vi "Sender UI.vi"(8 "Error In":errorcluster, 10 "Transmission Type":T1, 11 "Transmission Data":string(combo)) -> (0 "Error Out":errorcluster)   [LabVIEW 2020, in "Sender.lvclass"]
doc: "The VI allows user to select the type of data to be send to receiver and type of transmission"
uses:
  Sender.lvclass
  Controls/Queue Operation.ctl
  Controls/User Event Operations.ctl
  Controls/Messenger Data.ctl
  Communication/Communication.lvclass
  Data/Data.lvclass
  Controls/Class DVR Ref.ctl
  Controls/Type Class Ref.ctl
  Controls/Message Type.ctl
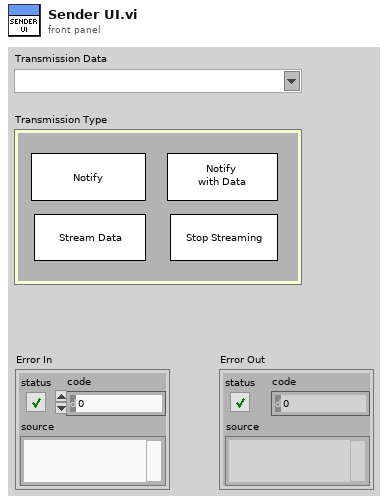
[diagram p1: front panel]
types:
  T1 = typedef "Message Type.ctl" = cluster{"Notify Only":bool, "Notify With Data":bool, "Stream Data":bool, "Stop Stream":bool}
  T2 = typedef "Messenger Data.ctl" = cluster{"Start Time":dbl, "Elapsed TIme":dbl, "Selected Data Type":string, "Selected Transmission Type":string, "Type DVR Ref":T3[], "Data DVR Ref":T4[], "Type DVR":refnum<data-value>, "Data DVR":refnum<data-value>, "Stream?":bool, "Wait Time":dbl}
  T3 = typedef "Type Class Ref.ctl" = cluster{"Class Name":string, "Class DVR Ref":refnum<data-value>}
  T4 = typedef "Class DVR Ref.ctl" = cluster{"Class DVR Ref":refnum<data-value>, "Class Name":string}
  T5 = typedef "User Event Operations.ctl" = enum16{"Obtain", "Generate", "Destroy"}
  T6 = typedef "Queue Operation.ctl" = enum16{"Create & Enqueue N", "Enqueue N", "Dequeue", "Enstack N", "Flush", "Release"}
  T7 = enum8{"Enabled", "Disabled", "Disabled and Grayed Out"}
  T8 = typedef "Queue Element.ctl" = cluster{"State":string, "Data":variant}
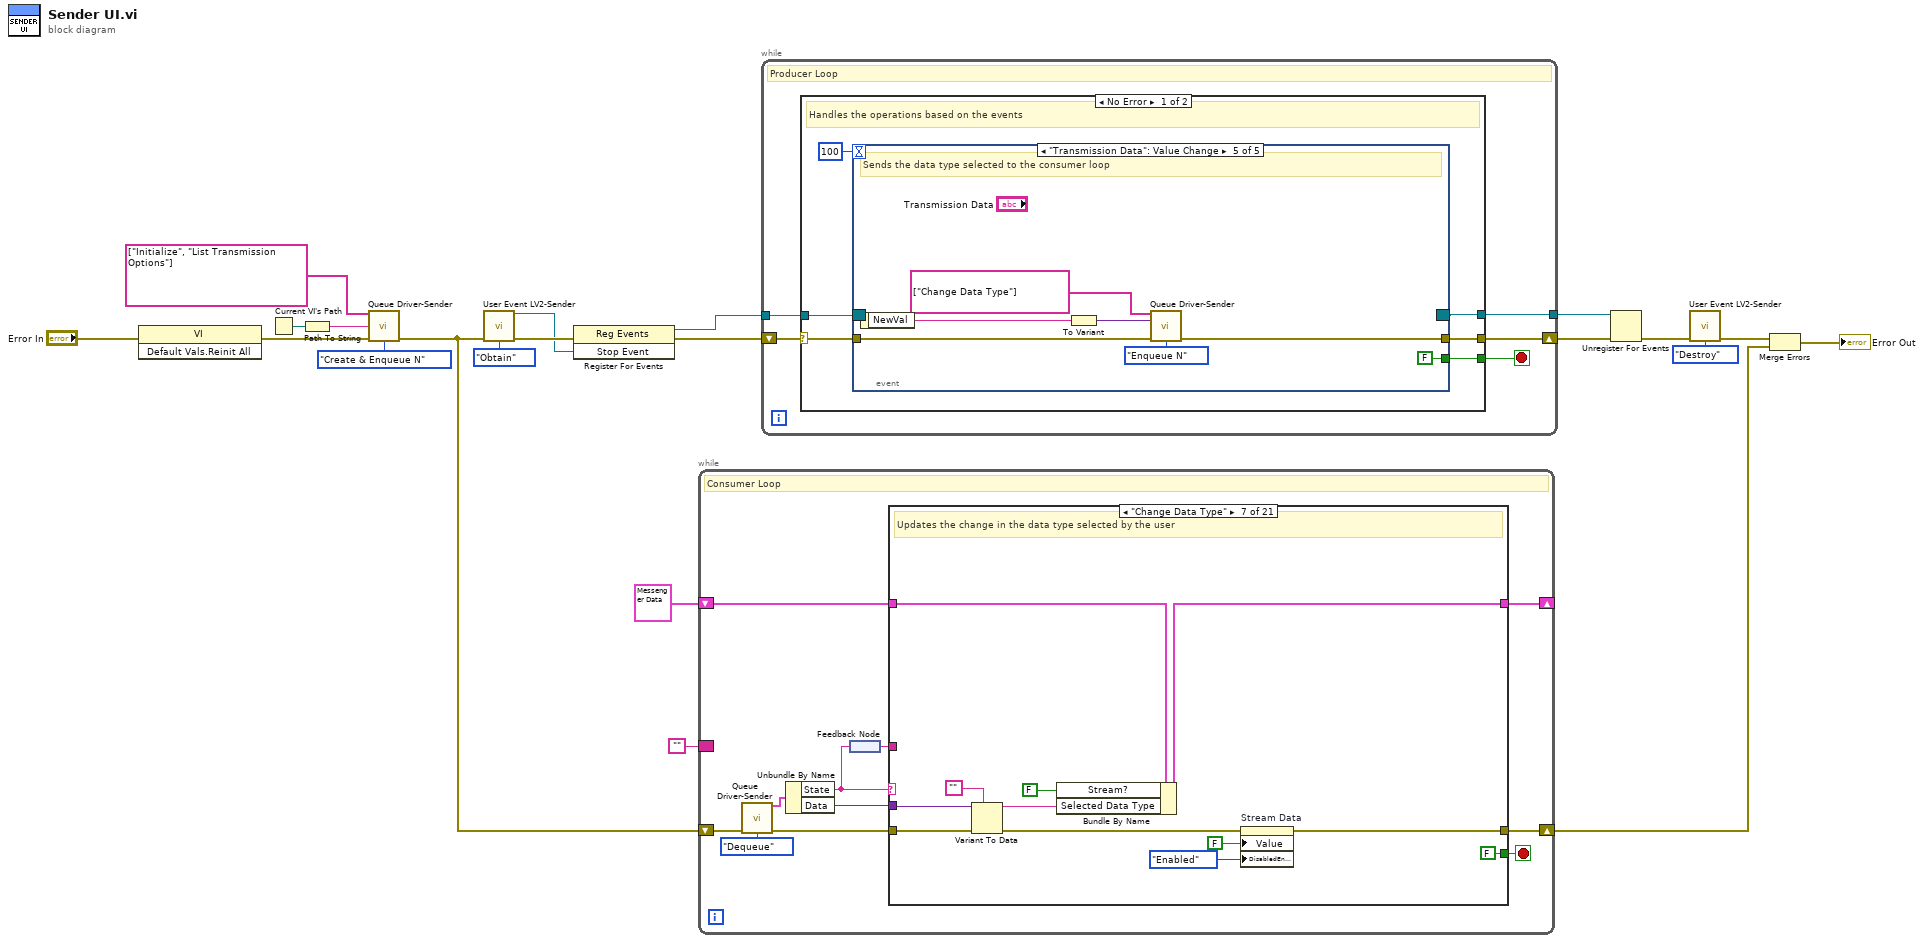
[diagram p0: block diagram]
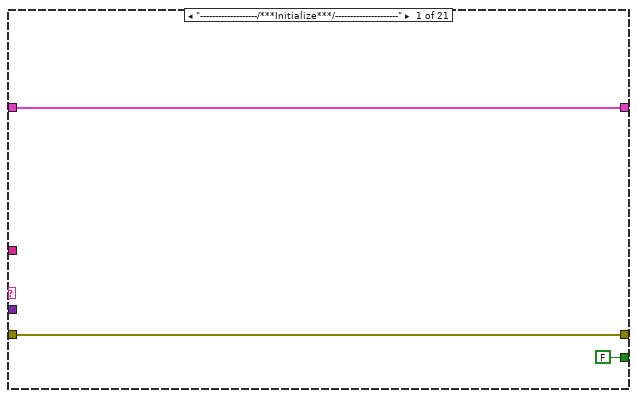
[diagram p2: hidden frame]
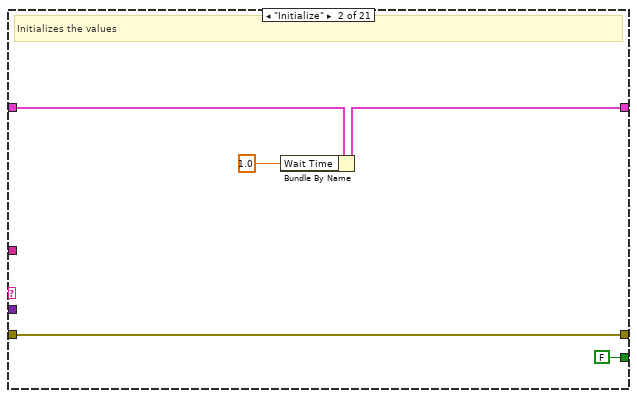
[diagram p3: hidden frame]
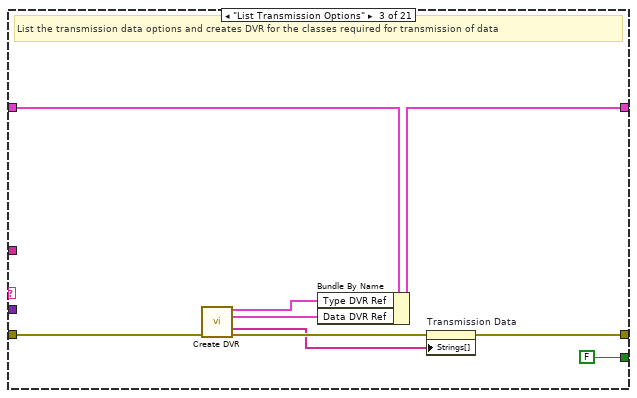
[diagram p4: hidden frame]
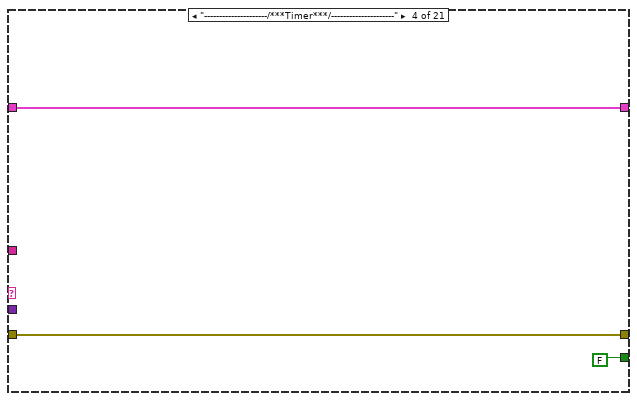
[diagram p5: hidden frame]
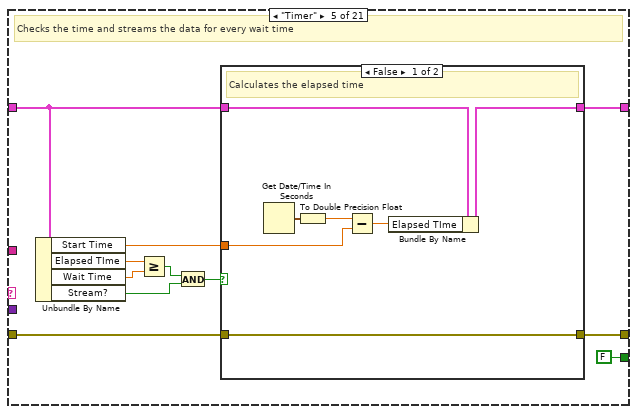
[diagram p6: hidden frame]
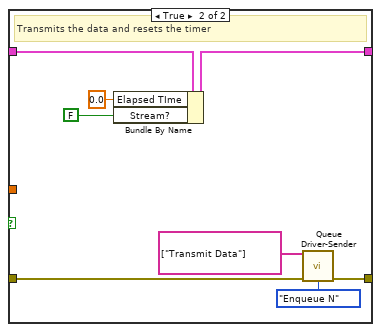
[diagram p7: hidden frame]
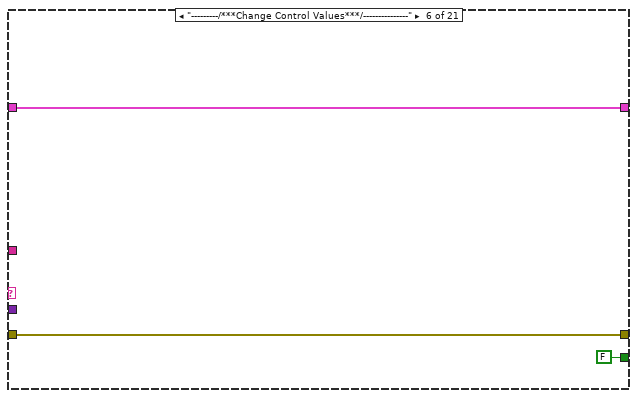
[diagram p8: hidden frame]
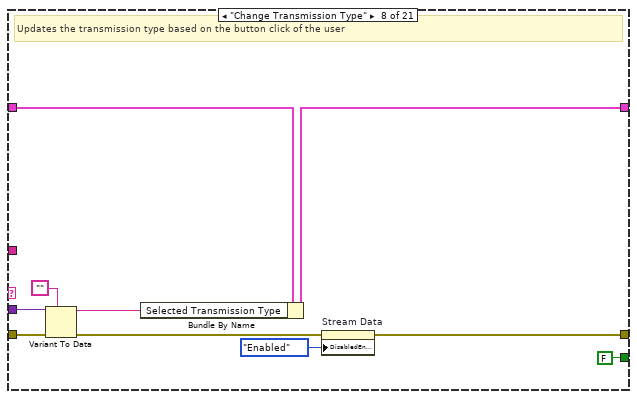
[diagram p9: hidden frame]
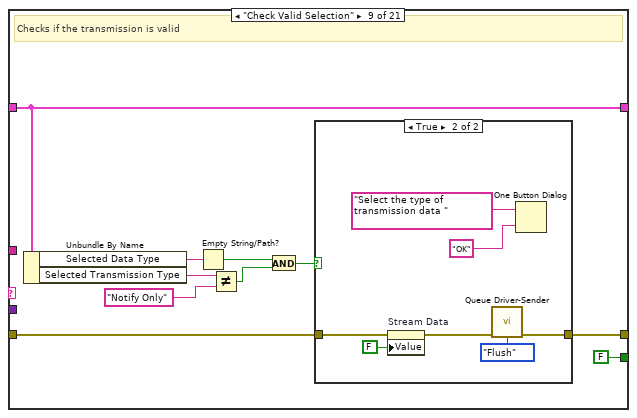
[diagram p10: hidden frame]
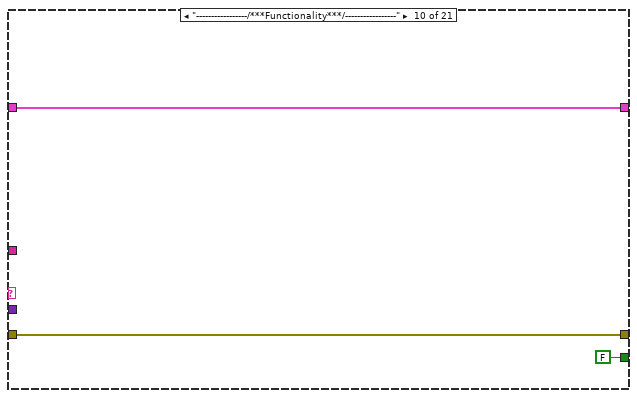
[diagram p12: hidden frame]
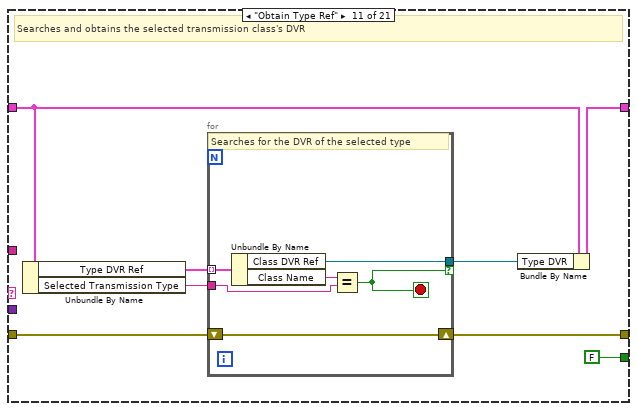
[diagram p13: hidden frame]
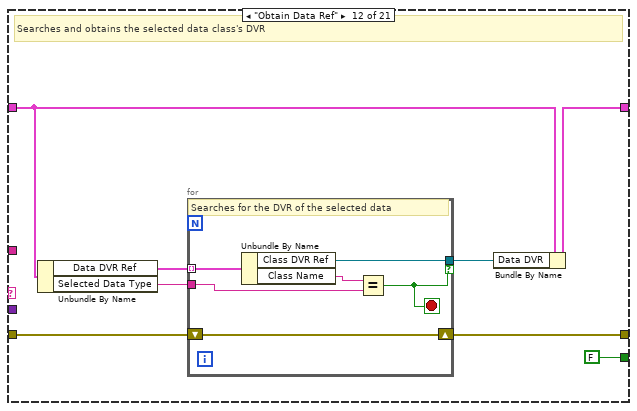
[diagram p14: hidden frame]
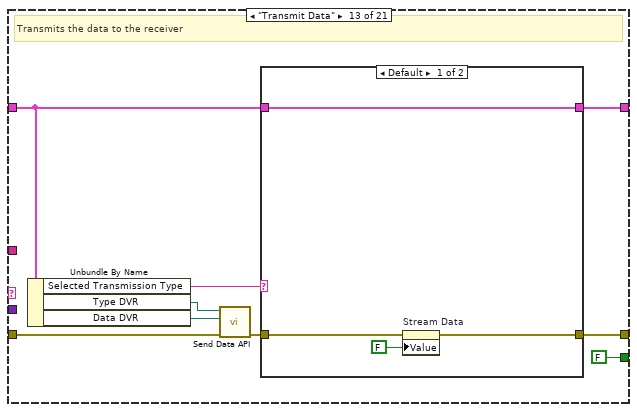
[diagram p15: hidden frame]
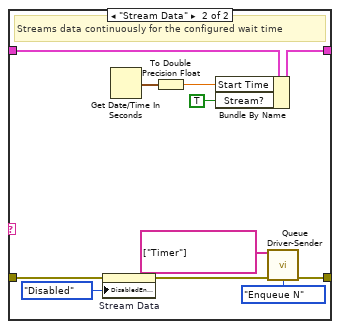
[diagram p16: hidden frame]
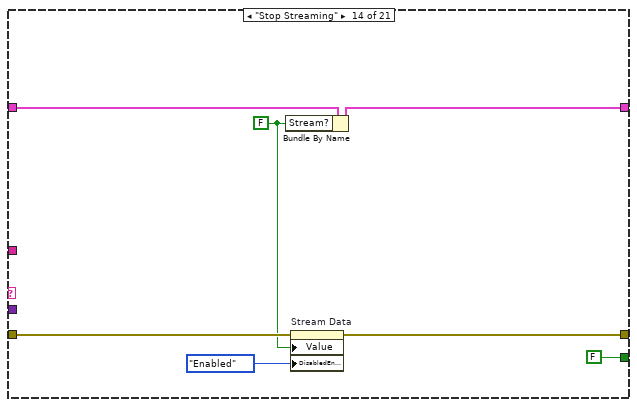
[diagram p17: hidden frame]
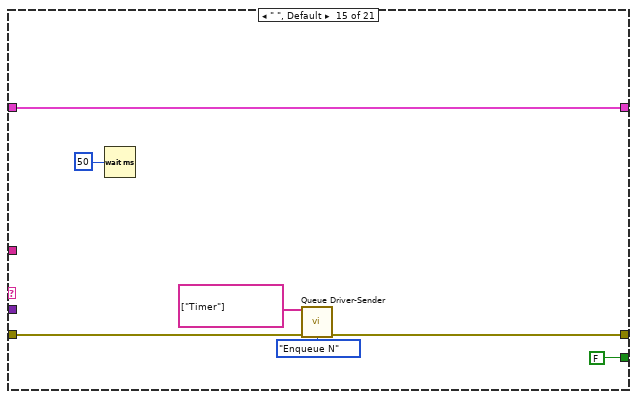
[diagram p18: hidden frame]
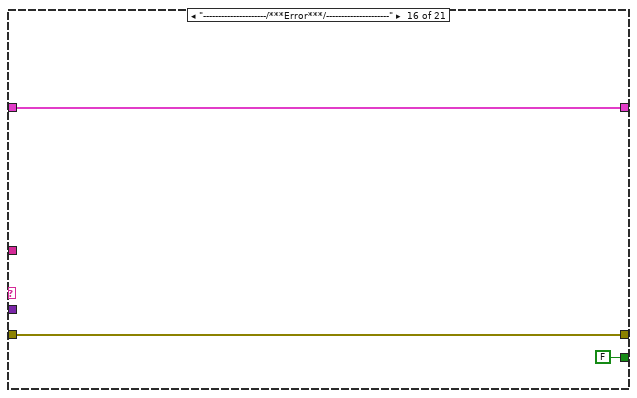
[diagram p19: hidden frame]
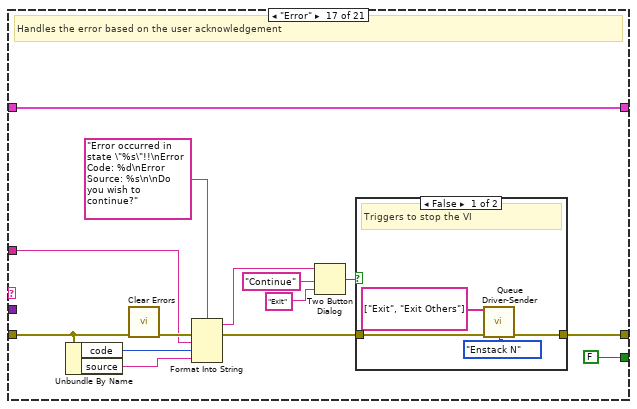
[diagram p20: hidden frame]
diagram:
  n1 = invoke class="VI" method="Default Vals.Reinit All"(error in="Error In") -> (error out=w1:errorcluster)  [unwired: 2 in, 2 out]
  n2 = Current VI's Path() -> (path=w3:path)
  n3 = Path To String(path=w3) -> (string=w2:string)
  n4 = call "Queue Driver-Sender.vi"("States[]"=string[] ["Initialize", "List Transmission Options"], "Queue Name"=w2, "Error In"=w1, "Queue Operation"=Queue_Operation."Create & Enqueue N") -> ("Error Out"=w13:errorcluster)  [unwired: 10 in, 1 out]
  n5 = call "User Event LV2-Sender.vi"("Error In"=w13, "Operation"=User_Event_Operations."Obtain") -> ("Stop Event"=w11:refnum<user-event>, "Error Out"=w15:errorcluster)  [unwired: 12 in]
  n6 = register-events(error in=w15, w11) -> (reference out=w10:refnum<event-registration>, error out=w12:errorcluster)  [unwired: 1 in]
  n7 = while {
    shift-right: [w31] -> w16
    shift-left: w13 -> [w32]
    border: "" -> [_]
    shift-right: [w22] -> _
    shift-left: T2 {"Start Time"=0.0, "Elapsed TIme"=0.0, "Selected Data Type"="", "Selected Transmission Type"="", "Type DVR Ref"=[], "Data DVR Ref"=[], "Type DVR"=refnum, "Data DVR"=refnum, "Stream?"=FALSE, "Wait Time"=0.0} -> [w23]
    stop <- w27 stop-if-true
    # "Consumer Loop"
    n8 = call "Queue Driver-Sender.vi"("Error In"=w32, "Queue Operation"=Queue_Operation."Dequeue") -> ("Dequeue Element"=w28:T8, "Error Out"=w30:errorcluster)  [unwired: 12 in]
    n9 = Unbundle By Name(w28) -> ("State"=w26:string, "Data"=w24:variant)
    n10 = feedback-in #1(w26) -> ()
    n11 = feedback #1() -> (w25:string)
    n12 = case shown="\"Change Data Type\"" w26 {
      tunnel: w30 -> [w35 w39 w49 w52 w63 w81 w93 w103 w113 w124 w132 w146 w161 w183 w190 w193 w199 w228 w236 w246 w255]
      tunnel: [w35 w39 w41 w52 w62 w81 w84 w95 w110 w124 w131 w145 w157 w179 w187 w193 w196 w215 w236 w242 w253] -> w31
      tunnel: [FALSE FALSE FALSE FALSE FALSE FALSE FALSE FALSE FALSE FALSE FALSE FALSE FALSE FALSE FALSE FALSE FALSE FALSE FALSE TRUE FALSE] -> w27
      tunnel: w25 -> [_ _ _ _ _ _ _ _ _ _ _ _ _ _ _ _ w197 _ _ _ _]
      tunnel: w24 -> [_ _ _ _ _ _ w88 w100 _ _ _ _ _ _ _ _ _ w220 _ _ _]
      tunnel: w23 -> [w33 w38 w47 w51 w60 w80 w90 w102 w111 w122 w130 w144 w156 w182 w188 w191 w194 w227 w234 w237 w254]
      tunnel: [w33 w37 w45 w51 w59 w80 w89 w98 w111 w122 w126 w140 w158 w181 w188 w191 w194 w227 w234 w237 w254] -> w22
      frame "-------------------/***Initialize***/---------------------" {
      }
      frame "Initialize" {
        # "Initializes the values"
        n13 = Bundle By Name(cluster=w38, "Wait Time"=1.0) -> (w37:T2)
      }
      frame "List Transmission Options" {
        # "List the transmission data options and creates DVR for the classes required for transmission of data"
        n14 = call "Create DVR.vi"("Error In"=w49) -> ("Communication DVR Refs"=w44:T3[], "Data Type DVR Refs"=w43:T4[], "Data Types"=w42:string[], "Error Out"=w46:errorcluster)  [unwired: 10 in, 1 out]
        n15 = Bundle By Name(cluster=w47, "Type DVR Ref"=w44, "Data DVR Ref"=w43) -> (w45:T2)
        n16 = property on="Transmission Data" class="CmbBox"(error in=w46, "Strings[]"=w42) -> (error out=w41:errorcluster)  [unwired: 1 in, 1 out]
      }
      frame "---------------------/***Timer***/---------------------" {
      }
      frame "Timer" {
        # "Checks the time and streams the data for every wait time"
        n17 = Unbundle By Name(w60) -> ("Start Time"=w61:dbl, "Elapsed TIme"=w57:dbl, "Wait Time"=w53:dbl, "Stream?"=w54:bool)
        n18 = Greater Or Equal?(x=w57, y=w53) -> (x >= y?=w56:bool)
        n19 = And(x=w56, y=w54) -> (x .and. y?=w55:bool)
        n20 = case shown="False" w55 {
          tunnel: w63 -> [w69 w71]
          tunnel: [w69 w77] -> w62
          tunnel: w61 -> [w64 _]
          tunnel: [w68 w74] -> w59
          tunnel: w60 -> [w70 w78]
          frame False {
            # "Calculates the elapsed time"
            n21 = Get Date/Time In Seconds() -> (seconds since 1Jan1904=w67:timestamp)
            n22 = To Double Precision Float(number=w67) -> (double precision float=w65:dbl)
            n23 = Subtract(x=w65, y=w64) -> (x-y=w66:dbl)
            n24 = Bundle By Name(cluster=w70, "Elapsed TIme"=w66) -> (w68:T2)
          }
          frame True {
            # "Transmits the data and resets the timer"
            n25 = Bundle By Name(cluster=w78, "Elapsed TIme"=0.0, "Stream?"=FALSE) -> (w74:T2)
            n26 = call "Queue Driver-Sender.vi"("States[]"=string[] ["Transmit Data"], "Error In"=w71, "Queue Operation"=Queue_Operation."Enqueue N") -> ("Error Out"=w77:errorcluster)  [unwired: 11 in, 1 out]
          }
        }
      }
      frame "---------/***Change Control Values***/---------------" {
      }
      frame "Change Data Type" {
        # "Updates the change in the data type selected by the user"
        n27 = Variant To Data(error in=w93, type="", Variant=w88) -> (data=w86:string, error out=w87:errorcluster)
        n28 = Bundle By Name(cluster=w90, "Stream?"=FALSE, "Selected Data Type"=w86) -> (w89:T2)
        n29 = property on="Stream Data" class="Bool (strict)"(error in=w87, "Value"=FALSE, "DisabledEnum"=T7."Enabled" ("Disabled")) -> (error out=w84:errorcluster)  [unwired: 1 in, 1 out]
      }
      frame "Change Transmission Type" {
        # "Updates the transmission type based on the button click of the user"
        n30 = Variant To Data(error in=w103, type="", Variant=w100) -> (data=w97:string, error out=w101:errorcluster)
        n31 = Bundle By Name(cluster=w102, "Selected Transmission Type"=w97) -> (w98:T2)
        n32 = property on="Stream Data" class="Bool (strict)"(error in=w101, "DisabledEnum"=T7."Enabled" ("Disabled")) -> (error out=w95:errorcluster)  [unwired: 1 in, 1 out]
      }
      frame "Check Valid Selection" {
        # "Checks if the transmission is valid"
        n33 = Unbundle By Name(w111) -> ("Selected Data Type"=w109:string, "Selected Transmission Type"=w107:string)
        n34 = Empty String/Path?(string/path=w109) -> (empty?=w106:bool)
        n35 = Not Equal?(x=w107, y="Notify Only") -> (x != y?=w105:bool)
        n36 = And(x=w106, y=w105) -> (x .and. y?=w104:bool)
        n37 = case shown="True" w104 {
          tunnel: w113 -> [w114 w121]
          tunnel: [w114 w118] -> w110
          frame False {
          }
          frame True {
            n38 = property on="Stream Data" class="Bool (strict)"(error in=w121, "Value"=FALSE) -> (error out=w116:errorcluster)  [unwired: 1 in, 1 out]
            n39 = call "Queue Driver-Sender.vi"("Error In"=w116, "Queue Operation"=Queue_Operation."Flush") -> ("Error Out"=w118:errorcluster)  [unwired: 12 in, 1 out]
            n40 = One Button Dialog(message="Select the type of transmission data ", button name ("OK")="OK") -> ()  [unwired: 1 out]
          }
        }
      }
      frame "-----------------/***Functionality***/-----------------" {
      }
      frame "Obtain Type Ref" {
        # "Searches and obtains the selected transmission class's DVR"
        n41 = Unbundle By Name(w130) -> ("Type DVR Ref"=w129:T3[], "Selected Transmission Type"=w128:string)
        n42 = for {
          shift-right: [w138] -> w131
          shift-left: w132 -> [w138]
          tunnel: w129 -> [w137] mode=indexing
          tunnel: w128 -> [w135]
          tunnel: [w134] -> w125 if=w133
          stop <- w133 stop-if-true
          # "Searches for the DVR of the selected type"
          n43 = Unbundle By Name(w137) -> ("Class DVR Ref"=w134:refnum<data-value>, "Class Name"=w136:string)
          n44 = Equal?(x=w136, y=w135) -> (x = y?=w133:bool)
        }
        n45 = Bundle By Name(cluster=w130, "Type DVR"=w125) -> (w126:T2)
      }
      frame "Obtain Data Ref" {
        # "Searches and obtains the selected data class's DVR"
        n46 = Unbundle By Name(w144) -> ("Data DVR Ref"=w143:T4[], "Selected Data Type"=w142:string)
        n47 = for {
          shift-right: [w152] -> w145
          shift-left: w146 -> [w152]
          tunnel: w143 -> [w151] mode=indexing
          tunnel: w142 -> [w148]
          tunnel: [w150] -> w139 if=w147
          stop <- w147 stop-if-true
          # "Searches for the DVR of the selected data"
          n48 = Unbundle By Name(w151) -> ("Class DVR Ref"=w150:refnum<data-value>, "Class Name"=w149:string)
          n49 = Equal?(x=w149, y=w148) -> (x = y?=w147:bool)
        }
        n50 = Bundle By Name(cluster=w144, "Data DVR"=w139) -> (w140:T2)
      }
      frame "Transmit Data" {
        # "Transmits the data to the receiver"
        n51 = Unbundle By Name(w156) -> ("Selected Transmission Type"=w155:string, "Type DVR"=w153:refnum<data-value>, "Data DVR"=w154:refnum<data-value>)
        n52 = call "Send Data API.vi"("Error In"=w161, "Data DVR"=w154, "Type DVR"=w153) -> ("Error Out"=w159:errorcluster)  [unwired: 7 in, 1 out]
        n53 = case shown="Default" w155 {
          tunnel: w159 -> [w164 w176]
          tunnel: [w165 w175] -> w158
          tunnel: [w163 w172] -> w157
          tunnel: w156 -> [w165 w169]
          frame Default {
            n54 = property on="Stream Data" class="Bool (strict)"(error in=w164, "Value"=FALSE) -> (error out=w163:errorcluster)  [unwired: 1 in, 1 out]
          }
          frame "Stream Data" {
            # "Streams data continuously for the configured wait time"
            n55 = property on="Stream Data" class="Bool (strict)"(error in=w176, "DisabledEnum"=T7."Disabled" ("Disabled")) -> (error out=w167:errorcluster)  [unwired: 1 in, 1 out]
            n56 = Get Date/Time In Seconds() -> (seconds since 1Jan1904=w173:timestamp)
            n57 = To Double Precision Float(number=w173) -> (double precision float=w174:dbl)
            n58 = Bundle By Name(cluster=w169, "Start Time"=w174, "Stream?"=TRUE) -> (w175:T2)
            n59 = call "Queue Driver-Sender.vi"("States[]"=string[] ["Timer"], "Error In"=w167, "Queue Operation"=Queue_Operation."Enqueue N") -> ("Error Out"=w172:errorcluster)  [unwired: 11 in, 1 out]
          }
        }
      }
      frame "Stop Streaming" {
        w178 = FALSE ("Stream?")
        n60 = Bundle By Name(cluster=w182, "Stream?"=w178) -> (w181:T2)
        n61 = property on="Stream Data" class="Bool (strict)"(error in=w183, "Value"=w178, "DisabledEnum"=T7."Enabled" ("Disabled")) -> (error out=w179:errorcluster)  [unwired: 1 in, 1 out]
      }
      frame " ", Default {
        n62 = Wait (ms)(milliseconds to wait=u32 50) -> ()  [unwired: 1 out]
        n63 = call "Queue Driver-Sender.vi"("States[]"=string[] ["Timer"], "Error In"=w190, "Queue Operation"=Queue_Operation."Enqueue N") -> ("Error Out"=w187:errorcluster)  [unwired: 11 in, 1 out]
      }
      frame "---------------------/***Error***/---------------------" {
      }
      frame "Error" {
        # "Handles the error based on the user acknowledgement"
        n64 = Unbundle By Name(w199) -> ("code"=w201:i32, "source"=w200:string)
        n65 = call <vilib>:"Clear Errors.vi"("error in (no error)"=w199) -> ("error out"=w206:errorcluster)  [unwired: 5 in, 1 out]
        n66 = Format Into String(format string="Error occurred in state \"%s\"!!\nError Code: %d\nError Source: %s\n\nDo you wish to continue?", error in=w206, w197, w201, w200) -> (resulting string=w204:string, error out=w198:errorcluster)  [unwired: 1 in]
        n67 = Two Button Dialog(message=w204, 1:"Exit" ("F button name (\"Cancel\")"), 2:"Continue" ("T button name (\"OK\")")) -> (T button?=w195:bool)
        n68 = case shown="False" w195 {
          tunnel: w198 -> [w211 w212]
          tunnel: [w210 w212] -> w196
          frame False {
            # "Triggers to stop the VI"
            n69 = call "Queue Driver-Sender.vi"("States[]"=string[] ["Exit", "Exit Others"], "Error In"=w211, "Queue Operation"=Queue_Operation."Enstack N") -> ("Error Out"=w210:errorcluster)  [unwired: 11 in, 1 out]
          }
          frame True {
          }
        }
      }
      frame "Producer Error" {
        n70 = Variant To Data(error in=w228, type=errorcluster {"status"=FALSE, "code"=0, "source"=""} ("error out"), Variant=w220) -> (data=w219:errorcluster, error out=w216:errorcluster)
        n71 = Unbundle By Name(w219) -> ("code"=w222:i32, "source"=w221:string)
        n72 = Format Into String(format string="Error occurred in producer loop\nError Code: %d\nError Source: %s\n\nDo you wish to continue?", error in=w216, w222, w221) -> (resulting string=w225:string, error out=w217:errorcluster)  [unwired: 1 in]
        n73 = Two Button Dialog(message=w225, 1:"Exit" ("F button name (\"Cancel\")"), 2:"Continue" ("T button name (\"OK\")")) -> (T button?=w214:bool)
        n74 = case shown="False" w214 {
          tunnel: w217 -> [w231 w233]
          tunnel: [w232 w233] -> w215
          frame False {
            n75 = call "Queue Driver-Sender.vi"("States[]"=string[] ["Exit"], "Error In"=w231, "Queue Operation"=Queue_Operation."Enstack N") -> ("Error Out"=w232:errorcluster)  [unwired: 11 in, 1 out]
          }
          frame True {
          }
        }
      }
      frame "----------------------/***Exit***/----------------------" {
      }
      frame "Exit" {
        # "Triggers the producer loop to stop and stops the consumer loop"
        n76 = call "User Event LV2-Sender.vi"("Event Name"="Stop Producer", "Error In"=w246, "Operation"=User_Event_Operations."Generate") -> ("Error Out"=w240:errorcluster)  [unwired: 11 in, 1 out]
        n77 = call "Queue Driver-Sender.vi"("Error In"=w240, "Queue Operation"=Queue_Operation."Flush") -> ("Error Out"=w244:errorcluster)  [unwired: 12 in, 1 out]
        n78 = call "Queue Driver-Sender.vi"("Error In"=w244, "Queue Operation"=Queue_Operation."Release") -> ("Error Out"=w242:errorcluster)  [unwired: 12 in, 1 out]
      }
      frame "Exit Others" {
        n79 = call "User Event LV2.vi"("Event Name"="", "Error In"=w255, "Operation"=User_Event_Operations."Generate") -> ("Error Out"=w250:errorcluster)  [unwired: 11 in, 1 out]
        n80 = call "User Event LV2-Receive.vi"("Event Name"="Stop", "Error In"=w250, "Operation"=User_Event_Operations."Generate") -> ("Error Out"=w253:errorcluster)  [unwired: 11 in, 1 out]
      }
    }
  }
  n81 = while {
    shift-right: [w258] -> w20
    shift-left: w12 -> [w259]
    tunnel: w10 -> [w257]
    tunnel: [w256] -> w8
    stop <- w260 stop-if-true
    # "Producer Loop"
    n82 = case shown="No Error" w259 {
      selector: w259 -> [w265 w304]
      tunnel: [w266 FALSE] -> w260
      tunnel: [w264 w307] -> w258
      tunnel: w257 -> [w262 _]
      tunnel: [w261 _] -> w256
      frame No Error {
        # "Handles the operations based on the events"
        n83 = event shown="[4] \"Transmission Data\": Value Change" {
          selector: w262 -> [_ _ _ _ _]
          dyn-events: [_ _ _ _ _] -> w261
          timeout: 100 -> [_ _ _ _ _]
          tunnel: [FALSE w270 FALSE FALSE FALSE] -> w266
          tunnel: w265 -> [w267 w272 w290 w295 w302]
          tunnel: [w267 w271 w289 w294 w300] -> w264
          event Timeout {
            # "Waits for any of the events to occur"
            n84 = event-data() -> ()  [unwired: 1 in, 3 out]
          }
          event User Event {
            # "Triggers to stop VI"
            n85 = event-data() -> ("State"=w269:string)  [unwired: 1 in]
            n86 = case shown="\"Stop Consumer\"" w269 {
              tunnel: w272 -> [w274 w276 w281]
              tunnel: [w274 w276 w279] -> w271
              tunnel: [FALSE TRUE FALSE] -> w270
              frame Default {
              }
              frame "Stop Producer" {
              }
              frame "Stop Consumer" {
                # "Initiates to stop the consumer loop"
                n87 = call "Queue Driver-Sender.vi"("States[]"=string[] ["Exit"], "Error In"=w281, "Queue Operation"=Queue_Operation."Enstack N") -> ("Error Out"=w279:errorcluster)  [unwired: 11 in, 1 out]
              }
            }
          }
          event Value Change {
            # "Initiates to start the data transmission"
            n88 = event-data() -> ("CtlRef"=w285:refnum<vi>)  [unwired: 1 in]
            n89 = property class="Bool"(reference=w285, error in=w290) -> (error out=w286:errorcluster, "Label.Text"=w283:string)  [unwired: 1 out]
            n90 = To Variant(anything=w283) -> (Variant=w282:variant)
            n91 = call "Queue Driver-Sender.vi"("States[]"=string[] ["Change Transmission Type", "Check Valid Selection", "Obtain Type Ref", "Obtain Data Ref", "Transmit Data"], "Data"=w282, "Error In"=w286, "Queue Operation"=Queue_Operation."Enqueue N") -> ("Error Out"=w289:errorcluster)  [unwired: 10 in, 1 out]
          }
          event Value Change {
            # "Stops the data streaming"
            n92 = event-data() -> ()  [unwired: 1 in, 1 out]
            n93 = call "Queue Driver-Sender.vi"("States[]"=string[] ["Stop Streaming"], "Error In"=w295, "Queue Operation"=Queue_Operation."Enqueue N") -> ("Error Out"=w294:errorcluster)  [unwired: 11 in, 1 out]
          }
          event "Transmission Data": Value Change {
            # "Sends the data type selected to the consumer loop"
            n94 = event-data() -> ("NewVal"=w299:string)  [unwired: 1 in]
            n95 = To Variant(anything=w299) -> (Variant=w297:variant)
            n96 = call "Queue Driver-Sender.vi"("States[]"=string[] ["Change Data Type"], "Data"=w297, "Error In"=w302, "Queue Operation"=Queue_Operation."Enqueue N") -> ("Error Out"=w300:errorcluster)  [unwired: 10 in, 1 out]
          }
        }
      }
      frame Error {
        # "Captures the error and sends to the consumer loop to handle"
        n97 = call <vilib>:"Clear Errors.vi"("error in (no error)"=w304) -> ("error out"=w308:errorcluster)  [unwired: 5 in, 1 out]
        n98 = To Variant(anything=w304) -> (Variant=w303:variant)
        n99 = call "Queue Driver-Sender.vi"("States[]"=string[] ["Exit Producer"], "Data"=w303, "Error In"=w308, "Queue Operation"=Queue_Operation."Enstack N") -> ("Error Out"=w307:errorcluster)  [unwired: 10 in, 1 out]
      }
    }
  }
  n100 = Unregister For Events(event registration refnum=w8, error in=w20) -> (error out=w9:errorcluster)
  n101 = call "User Event LV2-Sender.vi"("Error In"=w9, "Operation"=User_Event_Operations."Destroy") -> ("Error Out"=w7:errorcluster)  [unwired: 12 in, 1 out]
  n102 = Merge Errors(w7, w16) -> (→"Error Out":errorcluster)
